vi "Load Sound Player.vi"(11 "Select sound player:":T1 items=["Sound Card", "Sound Visualizer"]) -> (2 "error out":errorcluster, 3 "specific class reference":refnum<class "Sound Player.lvclass">)   [LabVIEW 2017, in "Sound Demo.lvclass"]
doc: "Dynamically load either Sound Visualizer\nor Sound Card.lvclass based on user input."
uses:
  Sound Demo.lvclass
  Select Sound Player.ctl
  Sound Player/Sound Player.lvclass
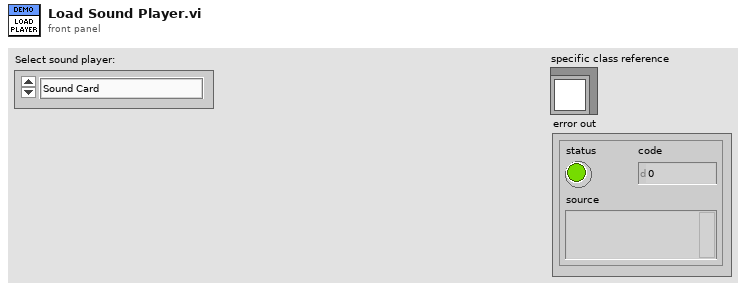
[diagram p1: front panel]
types:
  T1 = typedef "Sound Demo.lvclass/Select Sound Player.ctl" = u16
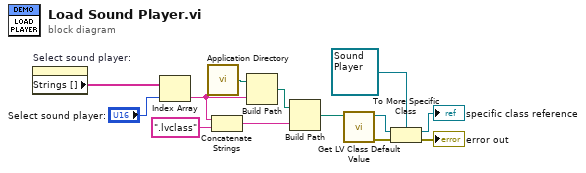
[diagram p0: block diagram]
diagram:
  n1 = property on="Select sound player:" class="Ring (strict)"() -> ("Strings []"=w13:string[])  [unwired: 2 in, 2 out]
  n2 = Index Array(array=w13, index="Select sound player:") -> (element=w10:string)
  n3 = call <vilib>:"Application Directory.vi"() -> ("Application Directory"=w11:path)
  n4 = Concatenate Strings(w10, ".lvclass" ("string")) -> (w7:string)
  n5 = Build Path(base path=w11, name or relative path=w10) -> (appended path=w8:path)
  n6 = Build Path(base path=w8, name or relative path=w7) -> (appended path=w6:path)
  n7 = call <vilib>:"Get LV Class Default Value.vi"("class path"=w6) -> ("error out"=w3:errorcluster, "object"=w5:refnum<class>)  [unwired: 9 in]
  n8 = To More Specific Class(target class=refnum<class "Sound Player.lvclass"> refnum ("Sound Player.lvclass"), reference=w5, error in=w3) -> (specific class reference=→"specific class reference":refnum<class "Sound Player.lvclass">, error out=→"error out":errorcluster)
